vi "1510 Distance Code.vi"(9 "Cannon Height in Inches":dbl, 10 "Target Height in Inches":dbl, 11 "Distance to Shoot In Feet":dbl) -> (3 "Wheel RPM":dbl)   [LabVIEW 2011]
panel:
  out "Wheel RPS":dbl
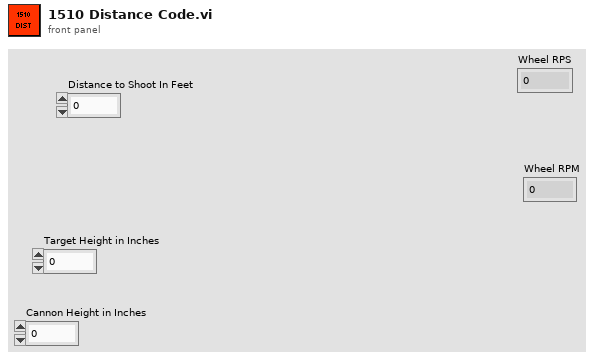
[diagram p1: front panel]
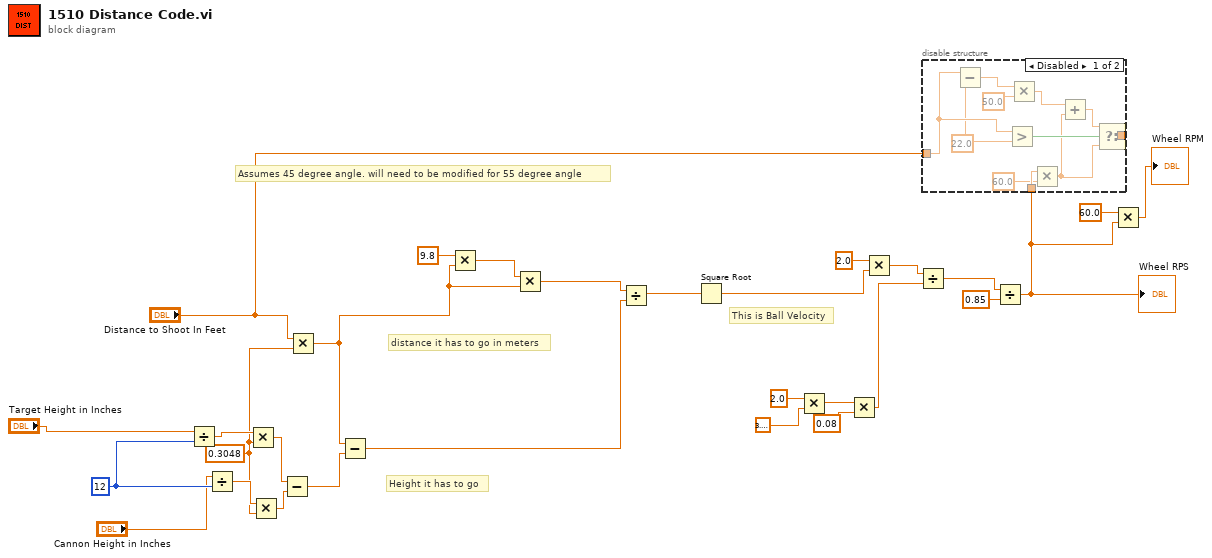
[diagram p0: block diagram]
diagram:
  w16 = 0.3048 ("y")
  w28 = 12
  # "distance it has to go in meters"
  # "Height it has to go"
  # "Assumes 45 degree angle. will need to be modified for 55 degree angle"
  # "This is Ball Velocity"
  n1 = Divide(x="Target Height in Inches", y=w28) -> (x/y=w26:dbl)
  n2 = Divide(x="Cannon Height in Inches", y=w28) -> (x/y=w23:dbl)
  n3 = Multiply(x=w26, y=w16) -> (x*y=w25:dbl)
  n4 = Multiply(x=w23, y=w16) -> (x*y=w24:dbl)
  n5 = Subtract(x=w25, y=w24) -> (x-y=w29:dbl)
  n6 = Multiply(x="Distance to Shoot In Feet", y=w16) -> (x*y=w17:dbl)
  n7 = Subtract(x=w17, y=w29) -> (x-y=w19:dbl)
  n8 = Multiply(x=9.8, y=w17) -> (x*y=w21:dbl)
  n9 = Multiply(x=w21, y=w17) -> (x*y=w20:dbl)
  n10 = Divide(x=w20, y=w19) -> (x/y=w18:dbl)
  n11 = Square Root(x=w18) -> (sqrt(x)=w14:dbl)
  n12 = Multiply(x=2.0, y=3.141592653589793) -> (x*y=w10:dbl)
  n13 = Multiply(x=w10, y=0.08) -> (x*y=w8:dbl)
  n14 = Multiply(x=2.0, y=w14) -> (x*y=w13:dbl)
  n15 = Divide(x=w13, y=w8) -> (x/y=w7:dbl)
  n16 = Divide(x=w7, y=0.85) -> (x/y=w4:dbl)
  "Wheel RPS" <- w4
  n17 = disable-structure shown="Disabled" {
    disable-tunnel: w4 -> [w40 _]
    disable-tunnel: "Distance to Shoot In Feet" -> [w37 _]
    disable-tunnel: [w31 _] -> _
    frame Disabled {
      w36 = 22.0 ("y")
      n18 = Subtract(x=w37, y=w36) -> (x-y=w35:dbl)
      n19 = Greater?(x=w37, y=w36) -> (0:w38:bool)
      n20 = Multiply(x=w35, y=50.0) -> (x*y=w33:dbl)
      n21 = Multiply(x=w40, y=60.0) -> (x*y=w30:dbl)
      n22 = Add(x=w33, y=w30) -> (x+y=w32:dbl)
      n23 = Select(t=w32, s=w38, f=w30) -> (s? t:f=w31:dbl)
    }
    frame Enabled {
    }
  }
  n24 = Multiply(x=60.0, y=w4) -> (x*y=→"Wheel RPM":dbl)
